vi "Configure Time Domain Gating.vi"(0 "VISA resource name":refnum<visa-resource-name>, 1 "Gating Function State (F: Disable)":bool, 2 "Setting Type (1: Start/Stop)":u16(ring)=1 items=["Center/Span", "Start/Stop"], 5 "Channel (1)":i32=1, 7 "Gate Type (0: Band-pass)":u16(ring) items=["Band-pass", "Notch"], 9 "Gate Shape (2: Normal Shape)":u16(ring)=2 items=["Maximum Shape", "Wide Shape", "Normal Shape", "Minimum Shape"], 11 "error in (no error)":errorcluster, 12 "Start / Center (0.0)":dbl format="%^.2e", 13 "Stop / Span (1.0E-8)":dbl=1e-08 format="%.2g") -> (4 "VISA resource name out":refnum<visa-resource-name>, 15 "error out":errorcluster)   [LabVIEW 2022 SP3, in "Agilent ENA Series.lvlib"]
doc: "Configures time domain gating."
uses:
  <instrlib>/Agilent ENA Series/Agilent ENA Series.lvlib
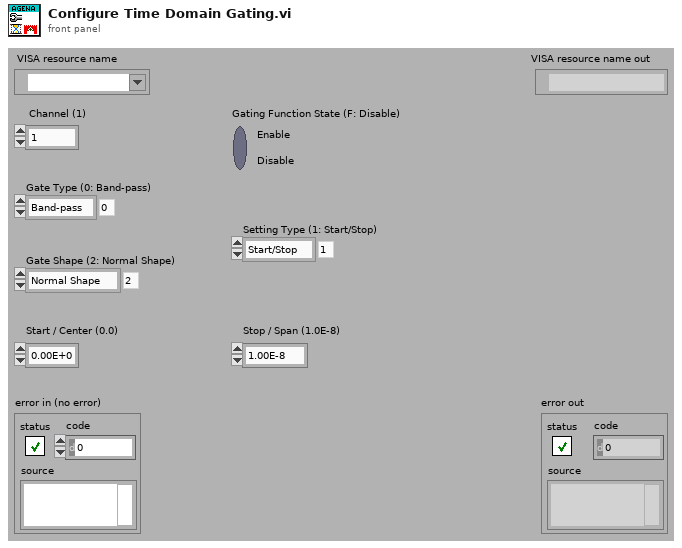
[diagram p1: front panel]
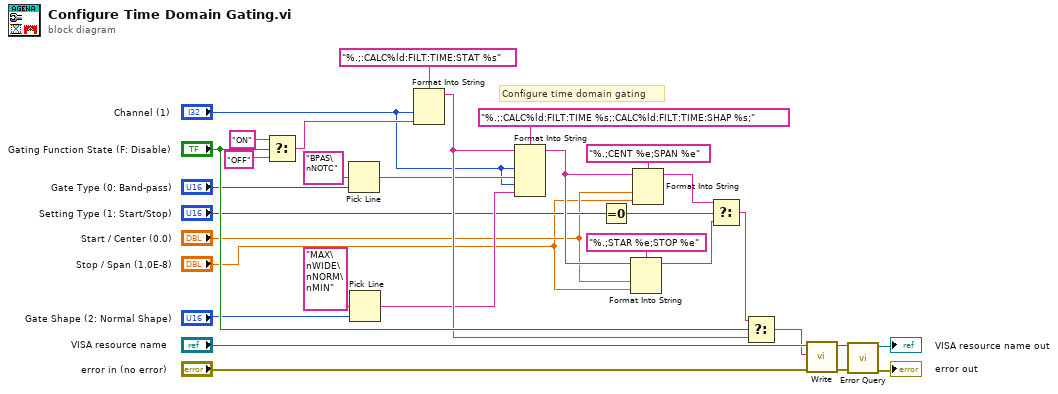
[diagram p0: block diagram]
diagram:
  # "Configure time domain gating"
  n1 = Select(t="ON", s="Gating Function State (F: Disable)", f="OFF") -> (s? t:f=w26:string)
  n2 = Pick Line(multi-line string="BPAS\nNOTC", line index="Gate Type (0: Band-pass)") -> (output string=w20:string)  [unwired: 1 in]
  n3 = Pick Line(multi-line string="MAX\nWIDE\nNORM\nMIN", line index="Gate Shape (2: Normal Shape)") -> (output string=w19:string)  [unwired: 1 in]
  n4 = Format Into String(format string="%.;:CALC%ld:FILT:TIME:STAT %s", "Channel (1)", w26) -> (resulting string=w23:string)  [unwired: 2 in, 1 out]
  n5 = Format Into String(format string="%.;:CALC%ld:FILT:TIME %s;:CALC%ld:FILT:TIME:SHAP %s;", initial string=w23, "Channel (1)", w20, "Channel (1)", w19) -> (resulting string=w16:string)  [unwired: 1 in, 1 out]
  n6 = Equal To 0?(x="Setting Type (1: Start/Stop)") -> (x = 0?=w15:bool)
  n7 = Format Into String(format string="%.;STAR %e;STOP %e", initial string=w16, "Start / Center (0.0)", "Stop / Span (1.0E-8)") -> (resulting string=w13:string)  [unwired: 1 in, 1 out]
  n8 = Format Into String(format string="%.;CENT %e;SPAN %e", initial string=w16, "Start / Center (0.0)", "Stop / Span (1.0E-8)") -> (resulting string=w14:string)  [unwired: 1 in, 1 out]
  n9 = Select(t=w14, s=w15, f=w13) -> (s? t:f=w12:string)
  n10 = Select(t=w12, s="Gating Function State (F: Disable)", f=w23) -> (s? t:f=w11:string)
  n11 = call <instrlib>:"Write.vi"("error in (no error)"="error in (no error)", "String ()"=w11, "VISA resource name"="VISA resource name") -> ("error out"=w3:errorcluster, "VISA resource name out"=w4:refnum<visa-resource-name>)  [unwired: 6 in, 1 out]
  n12 = call <instrlib>:"Error Query.vi"("error in (no error)"=w3, "VISA resource name"=w4) -> ("error out"=→"error out":errorcluster, "VISA resource name out"=→"VISA resource name out":refnum<visa-resource-name>)  [unwired: 6 in, 2 out]
